vi "Cinemática Directa.vi"(0 "t1":dbl, 1 "t2":dbl, 2 "L0":dbl, 3 "t3":dbl, 4 "L1":dbl, 5 "L2":dbl, 7 "L3":dbl) -> (20 "x":dbl, 24 "y":dbl, 27 "z":dbl)   [LabVIEW 2016]
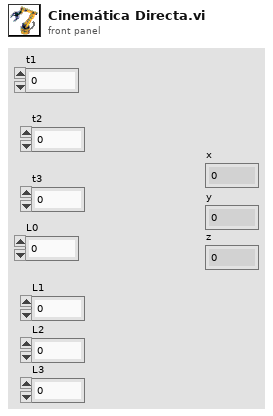
[diagram p1: front panel]
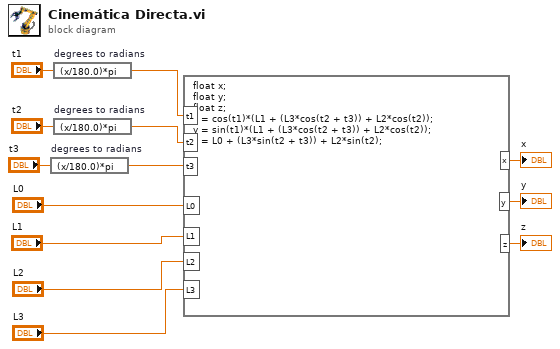
[diagram p0: block diagram]
diagram:
  n1 = expression code="(x/180.0)*pi" "degrees to radians"("t3") -> (w3:dbl)
  n2 = expression code="(x/180.0)*pi" "degrees to radians"("t1") -> (w6:dbl)
  n3 = expression code="(x/180.0)*pi" "degrees to radians"("t2") -> (w2:dbl)
  n4 = formula code="float x;\nfloat y;\nfloat z;\nx = cos(t1)*(L1 + (L3*cos(t2 + t3)) + L2*cos(t2));\ny = sin(t1)*(L1 + (L3*cos(t2 + t3)) + L2*cos(t2));\nz = L0 + (L3*sin(t2 + t3)) + L2*sin(t2);"("t1"=w6, "t2"=w2, "t3"=w3, "L1"="L1", "L2"="L2", "L3"="L3", "L0"="L0") -> ("x"=→"x":dbl, "y"=→"y":dbl, "z"=→"z":dbl)
